vi "Read connection reference.vi"(8 "error in (no error)":errorcluster, 11 "ODBC in":refnum<class "ADODB.lvclass">) -> (0 "error out":errorcluster, 2 "reference":T1, 3 "ODBC out":refnum<class "ADODB.lvclass">)   [LabVIEW 2020, in "ADODB.lvclass"]
uses:
  ADODB.lvclass
  <vilib>/addons/database/Connection.llb/Conn ObjectReference.ctl
  ADODB.lvclass/ADODB.ctl
  <vilib>/addons/database/NI_Database_API.lvlib
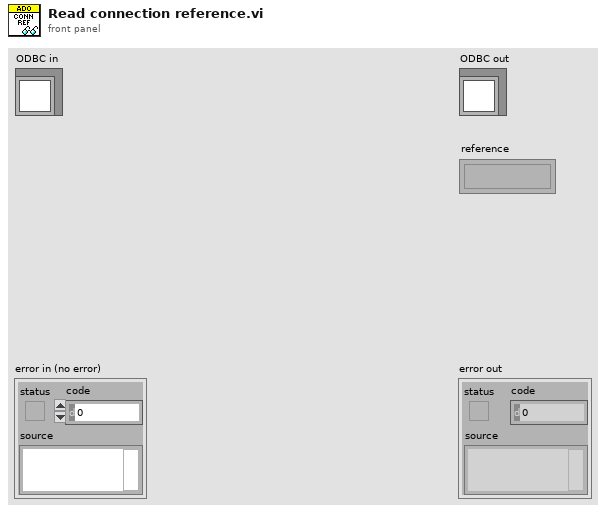
[diagram p1: front panel]
types:
  T1 = typedef "NI_Database_API.lvlib/Conn ObjectReference.ctl" = refnum<k1>
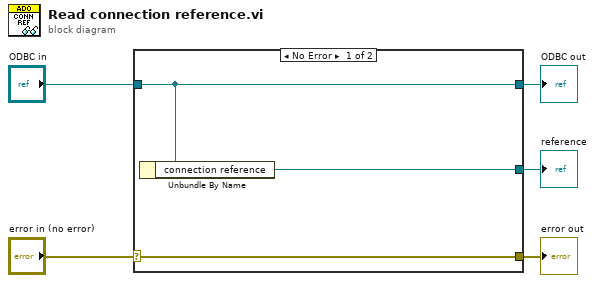
[diagram p0: block diagram]
diagram:
  n1 = case shown="No Error" "error in (no error)" {
    selector: "error in (no error)" -> [w8 w9]
    tunnel: [w8 w9] -> w4
    tunnel: [w7 w10] -> w2
    tunnel: "ODBC in" -> [w7 w10]
    tunnel: [w6 _] -> w1
    frame No Error {
      n2 = Unbundle By Name(w7) -> ("connection reference"=w6:T1)
    }
    frame Error {
    }
  }
  "error out" <- w4
  "ODBC out" <- w2
  "reference" <- w1
